vi "Stop.vi"(8 "Error In":errorcluster, 11 "reference in":refnum<class "Scope Simulated.lvclass">) -> (0 "Error Out":errorcluster, 3 "reference out":refnum<class "Scope Simulated.lvclass">)   [LabVIEW 2023, in "Scope Simulated.lvlib" / "Scope Simulated.lvclass"]
uses:
  Scope Simulated.lvclass
  Scope Simulated.lvclass/Scope Simulated.ctl
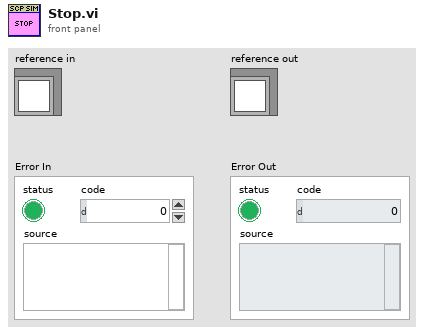
[diagram p1: front panel]
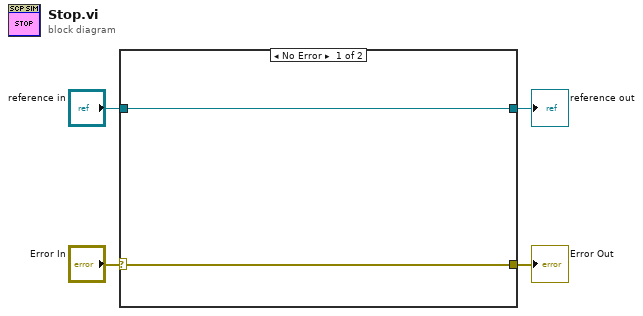
[diagram p0: block diagram]
diagram:
  n1 = case shown="No Error" "Error In" {
    selector: "Error In" -> [w5 w8]
    tunnel: [w5 w8] -> w3
    tunnel: [w6 w7] -> w1
    tunnel: "reference in" -> [w6 w7]
    frame No Error {
    }
    frame Error {
    }
  }
  "Error Out" <- w3
  "reference out" <- w1
